vi "Get Order-RPM Spectral Map (U8).vi"(6 "order range (auto)":T1 {"increment" format="%.2f"; "maximum" format="%.2f"; "minimum" format="%.2f"}, 7 "dB On (T)":bool=TRUE, 8 "error in (no error)":errorcluster, 9 "Gabor template":dbl[](array[numeric]) format="%.2f", 10 "sampling frequency [Hz]":dbl=1.0 format="%.2f", 11 "RefNum in":T2) -> (0 "error out":errorcluster, 1 "quantization info":cluster{"offset":dbl, "multiplier":dbl} {"multiplier" format="%.2f"; "offset" format="%.2f"}, 2 "spectral map":u8[][](array[numeric]), 3 "RefNum out":T2, 4 "order scale":cluster{"offset":dbl, "multiplier":dbl} {"multiplier" format="%.2f"; "offset" format="%.2f"}, 5 "rpm scale":cluster{"offset":dbl, "multiplier":dbl} {"multiplier" format="%.2f"; "offset" format="%.2f"})   [LabVIEW 2017, in "SoundVib_Gabor.lvlib"]
doc: "Generates an order-rpm spectral map of the data block referenced by <B>RefNum in</B>. You can use this polymorphic VI to return <B>spectral map</B> as a 2D array of double-precision, floating-point numbers or a 2D array of 8-bit unsigned integers. You must manually select the polymorphic instance to use. Use the DBL instance to obtain more accurate data. Use the U8 instance to reduce memory usage when the VI displays data."
uses:
  <vilib>/addons/Sound and Vibration/Order Analysis/Gabor Order Tracking/SoundVib_Gabor.lvlib
  <vilib>/addons/Sound and Vibration/Order Analysis/Ref Gabor Order Tracking/GT RefNum.ctl
  <resource>/sndvib.dll
panel:
  # "Get Order-RPM Spectral Map (U8)"
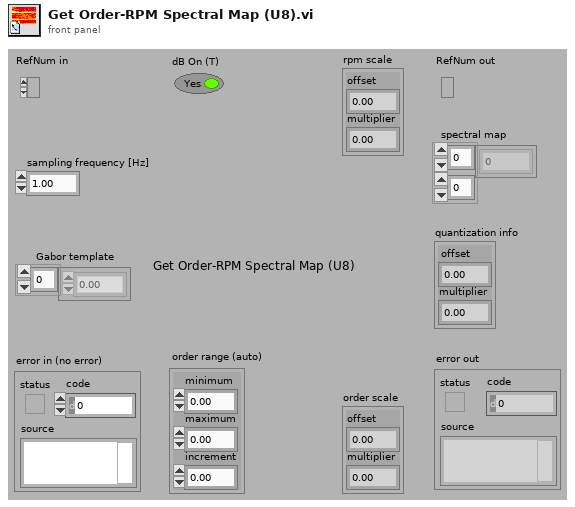
[diagram p1: front panel]
types:
  T1 = cluster{"minimum":dbl, "maximum":dbl, "increment":dbl}
  T2 = typedef "SoundVib_Gabor.lvlib/GT RefNum.ctl" = refnum<k1>
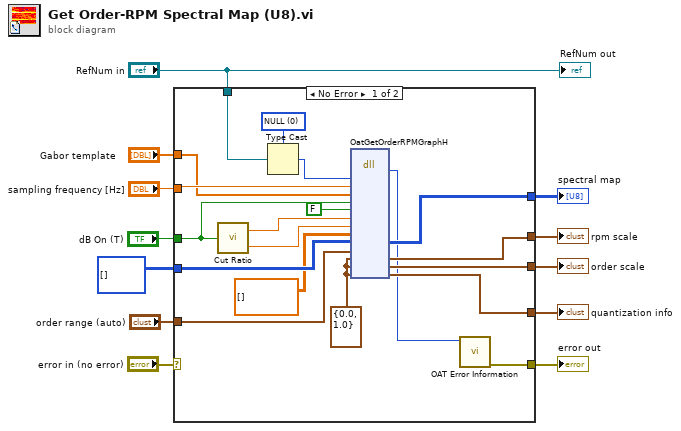
[diagram p0: block diagram]
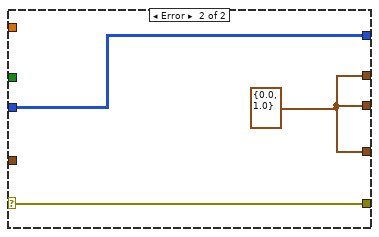
[diagram p2: hidden frame]
diagram:
  n1 = case shown="No Error" "error in (no error)" {
    selector: "error in (no error)" -> [_ w34]
    tunnel: [w31 w34] -> w5
    tunnel: "RefNum in" -> [w29 _]
    tunnel: [w25 w33] -> w2
    tunnel: [w16 w32] -> w3
    tunnel: [w24 w33] -> w4
    tunnel: [w26 w33] -> w12
    tunnel: "sampling frequency [Hz]" -> [w19 _]
    tunnel: "dB On (T)" -> [w21 _]
    tunnel: "Gabor template" -> [w18 _]
    tunnel: "order range (auto)" -> [w28 _]
    tunnel: u8[][] [] ("Graph") -> [w15 w32]
    frame No Error {
      w27 = cluster{"Z Min":dbl, "Z Step":dbl} {"Z Min"=0.0, "Z Step"=1.0}
      w30 = u32 0 items=["NULL"]
      n2 = call <vilib>:"Cut Ratio.vi"("dB On (T)"=w21) -> ("UpperCutRatio"=w22:dbl, "LowerCutRatio"=w23:dbl)
      n3 = Type Cast(type=w30, x=w29) -> (*(type *) &x=w20:u32)
      n4 = dll-call lib="C:/Program Files (x86)/National Instruments/LabVIEW 2017/resource/sndvib.*" fn="OatGetOrderRPMGraphH"("Ref In"=w20, "fs"=w19, "CntFreq"=w18, "bLogZ"=w21, "bGetDBL"=FALSE ("dB On (T)"), "uCutRatio"=w22, "dCutRatio"=w23, "DBLGraph"=dbl[][] [], "U8Graph"=w15, "OrderRange"=w28, "XScale"=w27, "YScale"=w27, "ZScale"=w27) -> ("return type"=w14:i32, "U8Graph"=w16:u8[][], "XScale"=w26:cluster{"Z Min":dbl, "Z Step":dbl}, "YScale"=w24:cluster{"Z Min":dbl, "Z Step":dbl}, "ZScale"=w25:cluster{"Z Min":dbl, "Z Step":dbl})  [unwired: 12 in, 2 out]
      n5 = call <vilib>:"OAT Error Information.vi"("error code"=w14) -> ("error out"=w31:errorcluster)  [unwired: 6 in]
    }
    frame Error {
      w33 = cluster{"Z Min":dbl, "Z Step":dbl} {"Z Min"=0.0, "Z Step"=1.0}
    }
  }
  "error out" <- w5
  "quantization info" <- w2
  "order scale" <- w4
  "rpm scale" <- w12
  "spectral map" <- w3
  "RefNum out" <- "RefNum in"
